vi "get_status_power.vi"(8 "error in (no error)":errorcluster, 11 "LightSourceMH110124MaiTai in":refnum<class "LightSourceMH110124MaiTai.lvclass">) -> (0 "error out":errorcluster, 2 "output power":dbl[unit], 3 "LightSourceMH110124MaiTai out":refnum<class "LightSourceMH110124MaiTai.lvclass">)   [LabVIEW 2010, in "LightSourceMH110124MaiTai.lvclass"]
uses:
  LightSourceMH110124MaiTai.lvclass
  LightSourceMH110124MaiTai.lvclass/LightSourceMH110124MaiTai.ctl
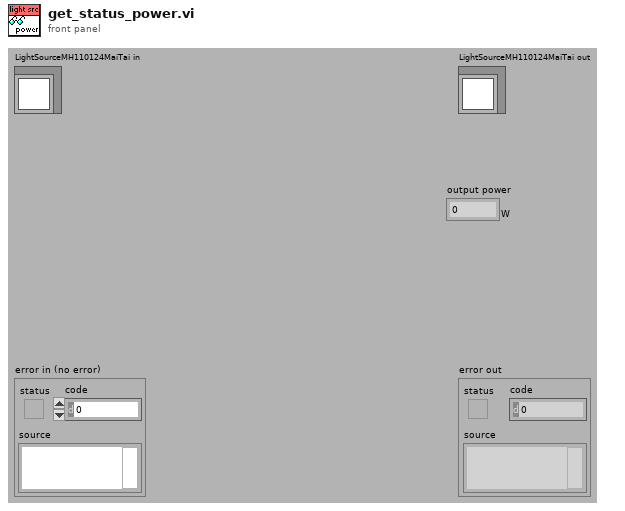
[diagram p1: front panel]
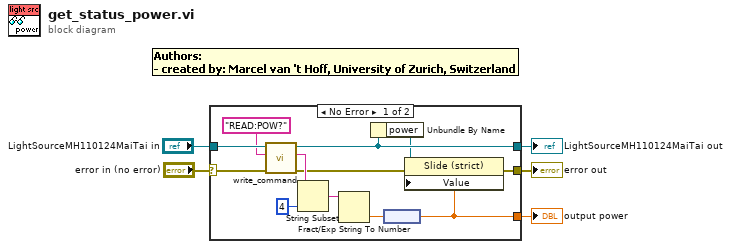
[diagram p0: block diagram]
diagram:
  n1 = case shown="No Error" "error in (no error)" {
    selector: "error in (no error)" -> [w16 w19]
    tunnel: [w9 w19] -> w2
    tunnel: [w11 w18] -> w3
    tunnel: "LightSourceMH110124MaiTai in" -> [w17 w18]
    tunnel: [w6 _] -> w1
    frame No Error {
      n2 = call-dynamic "write_command.vi"("error in (no error)"=w16, "string to write"="READ:POW?", "LightSourceMH110124MaiTai in"=w17) -> ("error out"=w10:errorcluster, "read string"=w14:string, "LightSourceMH110124MaiTai out"=w11:refnum<class "LightSourceMH110124MaiTai.lvclass">)  [unwired: 6 in]
      n3 = String Subset(string=w14, length (rest)=4 ("length (rest)")) -> (substring=w13:string)  [unwired: 1 in]
      n4 = Fract/Exp String To Number(string=w13) -> (number=w7:dbl)  [unwired: 3 in, 1 out]
      n5 = Unbundle By Name(w11) -> ("power"=w8:refnum<vi>)
      n6 = node(w7) -> (w6:dbl[unit])
      n7 = property class="Slide (strict)"(reference=w8, error in=w10, "Value"=w6) -> (error out=w9:errorcluster)  [unwired: 1 out]
    }
    frame Error {
    }
  }
  "error out" <- w2
  "LightSourceMH110124MaiTai out" <- w3
  "output power" <- w1
